vi "Temperature_value.vi"(2 "precision":i16=1, 3 "2nd byte":u8, 4 "1st byte":u8) -> (0 "Temperature string":string, 1 "Temperature value":dbl)   [LabVIEW 2012]
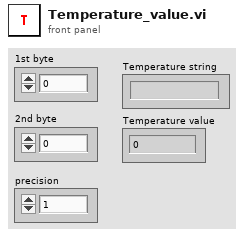
[diagram p1: front panel]
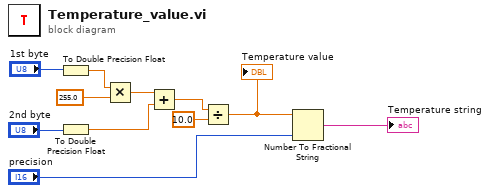
[diagram p0: block diagram]
diagram:
  n1 = To Double Precision Float(number="1st byte") -> (double precision float=w1:dbl)
  n2 = To Double Precision Float(number="2nd byte") -> (double precision float=w3:dbl)
  n3 = Multiply(x=w1, y=255.0) -> (x*y=w9:dbl)
  n4 = Add(x=w9, y=w3) -> (x+y=w8:dbl)
  n5 = Divide(x=w8, y=10.0) -> (x/y=w10:dbl)
  "Temperature value" <- w10
  n6 = Number To Fractional String(number=w10, precision (6)="precision") -> (F-format string=→"Temperature string":string)  [unwired: 2 in]
